vi "Handle Error.vi"(8 "error in (no error)":errorcluster, 11 "Service in":refnum<class "Service.lvclass">) -> (0 "error out":errorcluster, 2 "Stop Process":bool, 3 "Service out":refnum<class "Service.lvclass">)   [LabVIEW 2024, in "Ramses Framework.lvlib" / "Service.lvclass"]
uses:
  Service.lvclass
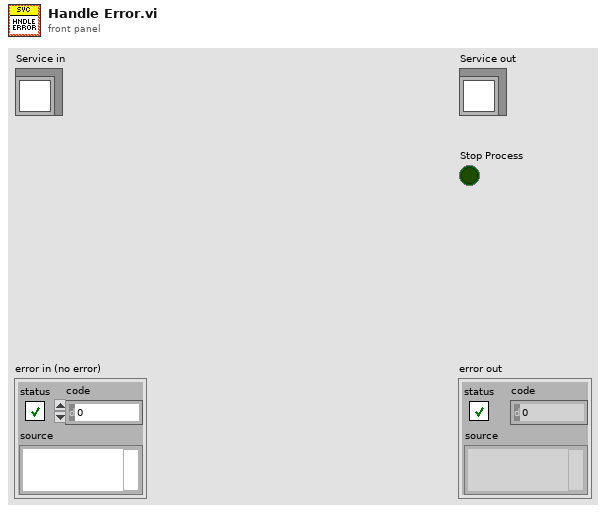
[diagram p1: front panel]
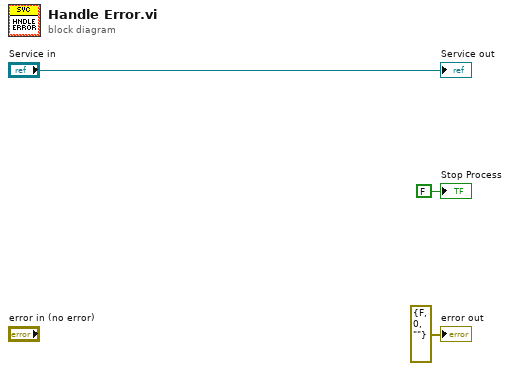
[diagram p0: block diagram]
diagram:
  "error out" <- errorcluster {"status"=FALSE, "code"=0, "source"=""} ("error out")
  "Service out" <- "Service in"
  "Stop Process" <- FALSE ("Stop Process")
